vi "Pre Launch Init.vi"(11 "XBox One Controller in":refnum<class "XBox One Controller.lvclass">) -> (0 "error out":errorcluster, 3 "XBox One Controller out":refnum<class "XBox One Controller.lvclass">)   [LabVIEW 2014, in "Xbox One Controller.lvlib" / "XBox One Controller.lvclass"]
doc: "(<B>Filename</B>: Actor Framework.lvlib:Actor.lvclass:Pre Launch Init.vi)\n\nDefines behavior that occurs after the Launch Actor method is invoked but before the actor's Actor Core method begins running.\n\nThe Pre Launch Init method is guaranteed to finish before the Launch Actor method returns to its caller and before the actor itself receives any messages. Any references that the Pre Launch Init method obtains are guaranteed to have the same lifetime as the actor itself. Any errors that the Pre Launch Init method returns will abort the launch.\n\nBy default, this method does nothing. A descendant class may override it to define behavior."
uses:
  XBox One Controller.lvclass
  Joystick/Joystick Class/Joystick.lvclass
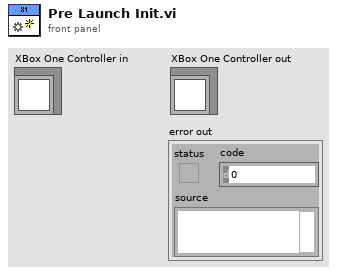
[diagram p1: front panel]
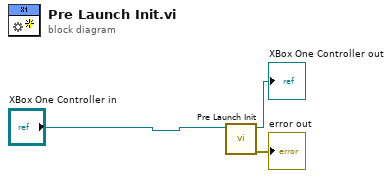
[diagram p0: block diagram]
diagram:
  n1 = call-parent "Pre Launch Init.vi"("System Actor in"="XBox One Controller in") -> ("error out"=→"error out":errorcluster, "System Actor out"=→"XBox One Controller out":refnum<class "XBox One Controller.lvclass">)  [unwired: 9 in]
